vi "Item Response.vi"(11 "Cache Item":T1) -> (0 "error out":errorcluster, 3 "Response":refnum<class "Response.lvclass">)   [LabVIEW 2020, in "HTTP Server.lvlib" / "Caching.lvclass"]
uses:
  Caching.lvclass
  Caching.lvclass/Caching.ctl
  lv-http-util/HTTP Utils/Response/Response.lvclass
  Cache Item.ctl
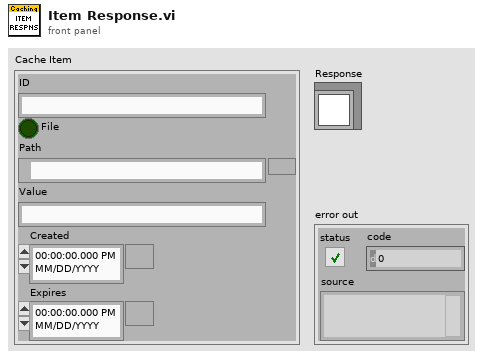
[diagram p1: front panel]
types:
  T1 = typedef "HTTP Server.lvlib/Caching.lvclass/Cache Item.ctl" = cluster{"ID":string, "File":bool, "Path":path, "Value":string, "Created":timestamp, "Expires":timestamp}
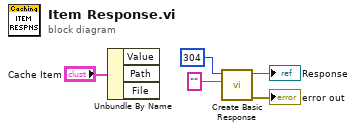
[diagram p0: block diagram]
diagram:
  n1 = Unbundle By Name("Cache Item") -> ()  [unwired: 3 out]
  n2 = call "Create Basic Response.vi"("Payload"="", "Status Code"=u16 304) -> ("error out"=→"error out":errorcluster, "Response out"=→"Response":refnum<class "Response.lvclass">)  [unwired: 8 in]
